vi "Update Class Instances.vi"(8 "error in (no error)":errorcluster, 9 "Step in":refnum<class "CallVIStep.lvclass">, 10 "Execution in":refnum<data-value>, 11 "VI Refnum in":refnum<vi>) -> (0 "error out":errorcluster, 1 "Step out":refnum<class "CallVIStep.lvclass">, 2 "Execution out":refnum<data-value>, 3 "VI Refnum out":refnum<vi>)   [LabVIEW 2015, in "CallVIStep.lvclass"]
uses:
  CallVIStep.lvclass
  Execution.lvclass
  Project.lvclass
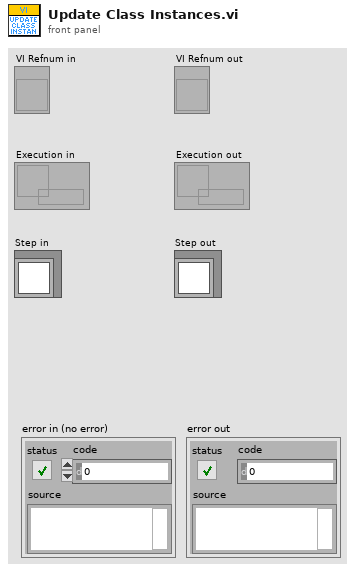
[diagram p1: front panel]
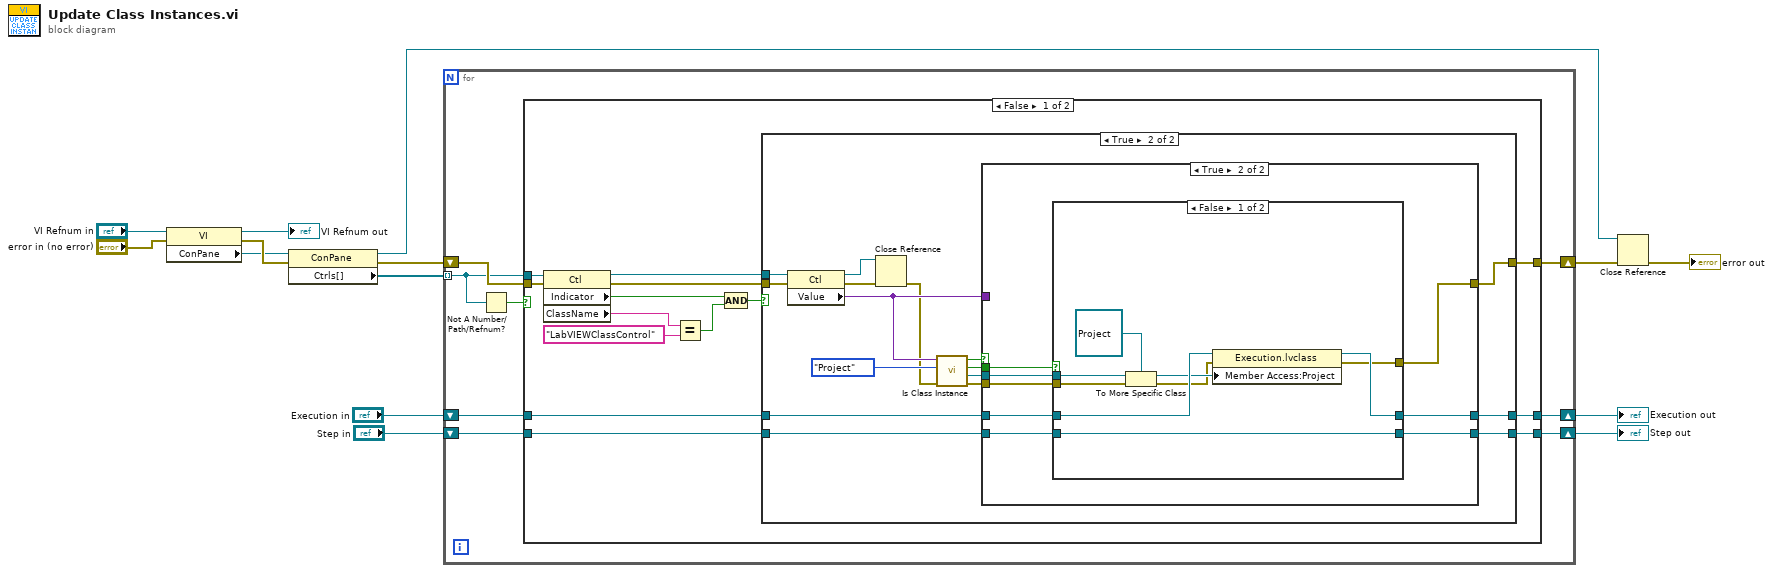
[diagram p0: block diagram]
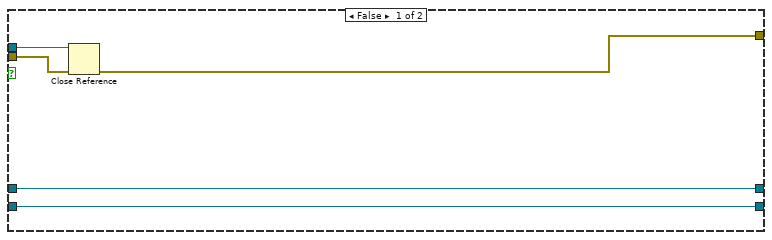
[diagram p2: hidden frame]
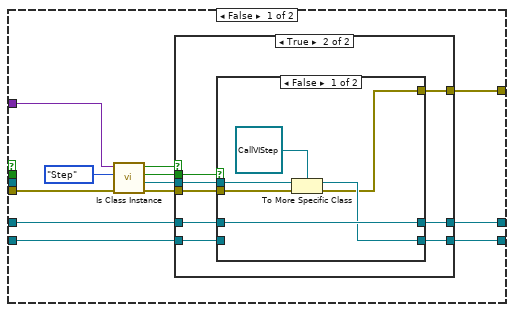
[diagram p3: hidden frame]
diagram:
  n1 = property class="VI"(reference="VI Refnum in", error in="error in (no error)") -> (reference out=→"VI Refnum out":refnum<vi>, error out=w13:errorcluster, "ConPane"=w11:refnum<vi>)
  n2 = property class="ConPane"(reference=w11, error in=w13) -> (reference out=w6:refnum<vi>, error out=w14:errorcluster, "Ctrls[]"=w12:refnum<vi>[])
  n3 = for {
    tunnel: w12 -> [w20] mode=indexing
    shift-right: [w21] -> w7
    shift-left: w14 -> [w22]
    shift-right: [w16] -> w2
    shift-left: "Step in" -> [w18]
    shift-right: [w15] -> w1
    shift-left: "Execution in" -> [w17]
    n4 = Not A Number/Path/Refnum?(number/path/refnum=w20) -> (NaN/Path/Refnum?=w19:bool)
    n5 = case shown="False" w19 {
      tunnel: w22 -> [w36 w112]
      tunnel: [w28 w112] -> w21
      tunnel: w20 -> [w27 _]
      tunnel: w18 -> [w26 w110]
      tunnel: w17 -> [w24 w111]
      tunnel: [w25 w110] -> w16
      tunnel: [w23 w111] -> w15
      frame False {
        n6 = property class="Ctl"(reference=w27, error in=w36) -> (reference out=w34:refnum<vi>, error out=w29:errorcluster, "Indicator"=w33:bool, "ClassName"=w31:string)
        n7 = Equal?(x=w31, y="LabVIEWClassControl") -> (x = y?=w32:bool)
        n8 = Compound Arithmetic op=AND(w33, w32) -> (w35:bool)
        n9 = case shown="True" w35 {
          tunnel: w34 -> [w41 w57]
          tunnel: w29 -> [w40 w56]
          tunnel: [w39 w42] -> w28
          tunnel: w26 -> [w37 w51]
          tunnel: [w37 w50] -> w25
          tunnel: w24 -> [w38 w49]
          tunnel: [w38 w46] -> w23
          frame False {
            n10 = Close Reference(reference=w41, error in (no error)=w40) -> (error out=w39:errorcluster)
          }
          frame True {
            n11 = property class="Ctl"(reference=w57, error in=w56) -> (reference out=w45:refnum<vi>, error out=w44:errorcluster, "Value"=w52:variant)
            n12 = Close Reference(reference=w45, error in (no error)=w44) -> (error out=w43:errorcluster)
            n13 = call "Is Class Instance.vi"("error in (no error)"=w43, "Class Type"=enum16{"Project", "Execution", "Step"}."Project", "Control Value"=w52) -> ("error out"=w54:errorcluster, "Class Instance"=w47:refnum<class>, "Is Default Value"=w48:bool, "Is Class Instance"=w55:bool)  [unwired: 5 in]
            n14 = case shown="True" w55 {
              tunnel: w54 -> [w58 w94]
              tunnel: [w67 w90] -> w42
              tunnel: w52 -> [w69 _]
              tunnel: w51 -> [w68 w92]
              tunnel: [w66 w91] -> w50
              tunnel: w49 -> [w65 w95]
              tunnel: w48 -> [_ w97]
              tunnel: w47 -> [_ w96]
              tunnel: [w64 w93] -> w46
              frame False {
                n15 = call "Is Class Instance.vi"("error in (no error)"=w58, "Class Type"=enum16{"Project", "Execution", "Step"}."Step", "Control Value"=w69) -> ("error out"=w61:errorcluster, "Class Instance"=w59:refnum<class>, "Is Default Value"=w60:bool, "Is Class Instance"=w62:bool)  [unwired: 5 in]
                n16 = case shown="True" w62 {
                  tunnel: w61 -> [w72 w74]
                  tunnel: w68 -> [w71 w79]
                  tunnel: [w72 w73] -> w67
                  tunnel: w60 -> [_ w80]
                  tunnel: w59 -> [_ w75]
                  tunnel: [w71 w78] -> w66
                  tunnel: w65 -> [w70 w77]
                  tunnel: [w70 w76] -> w64
                  frame False {
                  }
                  frame True {
                    n17 = case shown="False" w80 {
                      tunnel: w79 -> [_ w89]
                      tunnel: [w83 w89] -> w78
                      tunnel: w77 -> [w84 w88]
                      tunnel: [w84 w88] -> w76
                      tunnel: w75 -> [w86 _]
                      tunnel: w74 -> [w85 w87]
                      tunnel: [w81 w87] -> w73
                      frame False {
                        n18 = To More Specific Class(target class=refnum<class "CallVIStep.lvclass"> refnum ("CallVIStep.lvclass"), reference=w86, error in=w85) -> (specific class reference=w83:refnum<class "CallVIStep.lvclass">, error out=w81:errorcluster)
                      }
                      frame True {
                      }
                    }
                  }
                }
              }
              frame True {
                n19 = case shown="False" w97 {
                  tunnel: w96 -> [w105 _]
                  tunnel: w95 -> [w106 w108]
                  tunnel: w94 -> [w104 w109]
                  tunnel: [w100 w108] -> w93
                  tunnel: [w99 w109] -> w90
                  tunnel: w92 -> [w98 w107]
                  tunnel: [w98 w107] -> w91
                  frame False {
                    n20 = To More Specific Class(target class=refnum<class "Project.lvclass"> refnum ("Project.lvclass"), reference=w105, error in=w104) -> (specific class reference=w102:refnum<class "Project.lvclass">, error out=w101:errorcluster)
                    n21 = property class="Execution.lvclass"(reference=w106, error in=w101, "Member Access:Project"=w102) -> (reference out=w100:refnum<data-value>, error out=w99:errorcluster)
                  }
                  frame True {
                  }
                }
              }
            }
          }
        }
      }
      frame True {
      }
    }
  }
  "Step out" <- w2
  "Execution out" <- w1
  n22 = Close Reference(reference=w6, error in (no error)=w7) -> (error out=→"error out":errorcluster)
